vi "值已改变(I16 Array).vi"(1 "初始化":bool, 3 "输入数据":i32[](array[numeric])) -> (0 "已更改":bool)   [LabVIEW 2012]
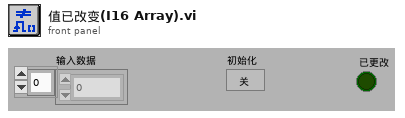
[diagram p1: front panel]
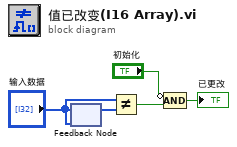
[diagram p0: block diagram]
diagram:
  n1 = feedback-in #1("输入数据") -> ()
  n2 = feedback #1("输入数据") -> (w5:i32[])
  n3 = Not Equal?(x="输入数据", y=w5) -> (x != y?=w4:bool)
  n4 = Compound Arithmetic op=AND(invert "初始化", w4) -> (→"已更改":bool)
